vi "read_attributes.vi"(8 "error in (no error)":errorcluster, 11 "AdaBoostRegressor in":refnum<class "AdaBoostRegressor.lvclass">) -> (0 "error out":errorcluster, 2 "attributes":T1, 3 "AdaBoostRegressor out":refnum<class "AdaBoostRegressor.lvclass">)   [LabVIEW 2020, in "AdaBoostRegressor.lvclass"]
uses:
  AdaBoostRegressor.lvclass
  Controls/adaboostregressor_attributes.ctl
  AdaBoostRegressor.lvclass/AdaBoostRegressor.ctl
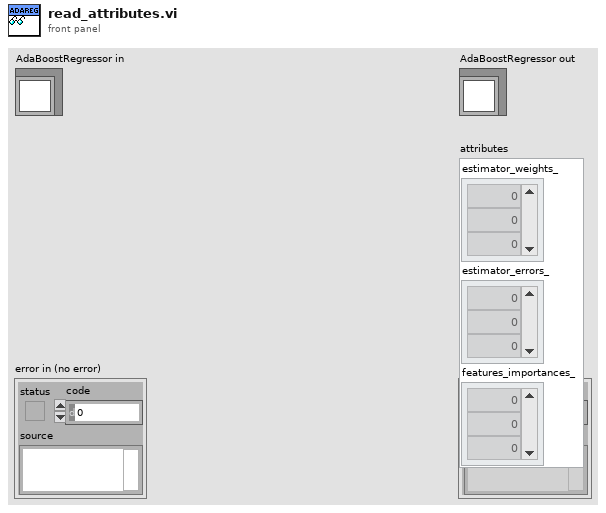
[diagram p1: front panel]
types:
  T1 = typedef "adaboostregressor_attributes.ctl" = cluster{"estimator_weights_":dbl[], "estimator_errors_":dbl[], "features_importances_":dbl[]}
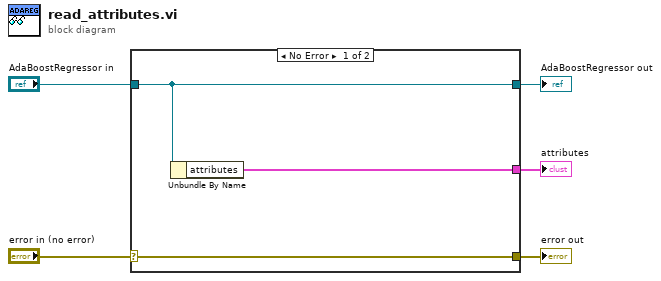
[diagram p0: block diagram]
diagram:
  n1 = case shown="No Error" "error in (no error)" {
    selector: "error in (no error)" -> [w8 w9]
    tunnel: [w8 w9] -> w4
    tunnel: [w7 w10] -> w2
    tunnel: "AdaBoostRegressor in" -> [w7 w10]
    tunnel: [w6 _] -> w1
    frame No Error {
      n2 = Unbundle By Name(w7) -> ("attributes"=w6:T1)
    }
    frame Error {
    }
  }
  "error out" <- w4
  "AdaBoostRegressor out" <- w2
  "attributes" <- w1
